vi "L10.vi"() -> ()   [LabVIEW 2012]
panel:
  out "sum":i64
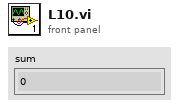
[diagram p1: front panel]
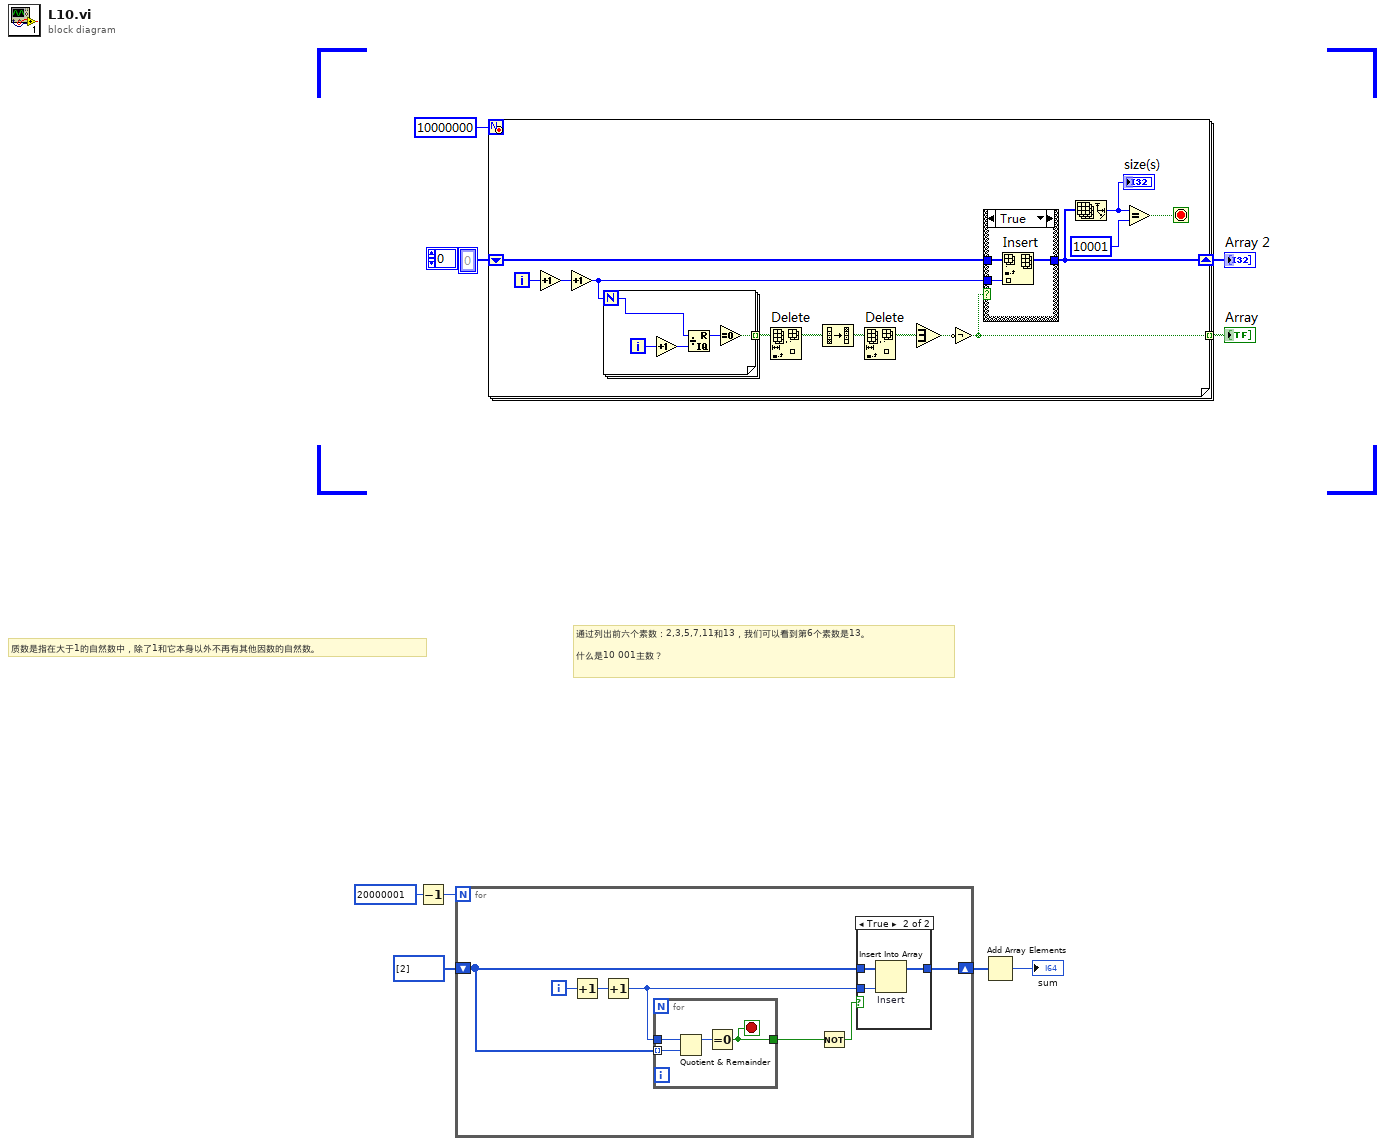
[diagram p0: block diagram]
diagram:
  # "通过列出前六个素数：2,3,5,7,11和13，我们可以看到第6个素数是13。\n\n什么是10 001主数？"
  # "质数是指在大于1的自然数中，除了1和它本身以外不再有其他因数的自然数。"
  n1 = Decrement(x=20000001) -> (x-1=w1:i32)
  n2 = for {
    N: w1 -> [_]
    shift-right: [w9] -> w2
    shift-left: i64[] [2] -> [w8]
    i -> [w12]
    n3 = Increment(x=w12) -> (x+1=w11:i32)
    n4 = Increment(x=w11) -> (x+1=w6:i32)
    n5 = for {
      tunnel: [w18] -> w7
      tunnel: w8 -> [w19] mode=indexing
      tunnel: w6 -> [w17]
      stop <- w18 stop-if-true
      n6 = Quotient & Remainder(x=w17, y=w19) -> (x-y*floor(x/y)=w20:i64)  [unwired: 1 out]
      n7 = Equal To 0?(x=w20) -> (x = 0?=w18:bool)
    }
    n8 = Not(x=w7) -> (.not. x?=w10:bool)
    n9 = case shown="True" w10 {
      tunnel: w8 -> [w13 w16]
      tunnel: [w13 w15] -> w9
      tunnel: w6 -> [_ w14]
      frame False {
      }
      frame True {
        n10 = Insert Into Array "Insert"(array=w16, new element=w14) -> (w15:i64[])  [unwired: 1 in]
      }
    }
  }
  n11 = Add Array Elements(numeric array=w2) -> (sum=→"sum":i64)
